vi "ble_evt_attclient_attribute_value.vi"(8 "error in (no error)":errorcluster, 11 "COM Bluegiga in":refnum<visa-resource-name>) -> (0 "error out":errorcluster, 1 "header_and_payload":u8[](array[numeric]), 2 "payload":u8[](array[numeric]), 3 "COM Bluegiga out":refnum<visa-resource-name>, 4 "attribute value":u8[](array[numeric]))   [LabVIEW 2013]
uses:
  type_def/message_class.ctl
  type_def/message_type.ctl
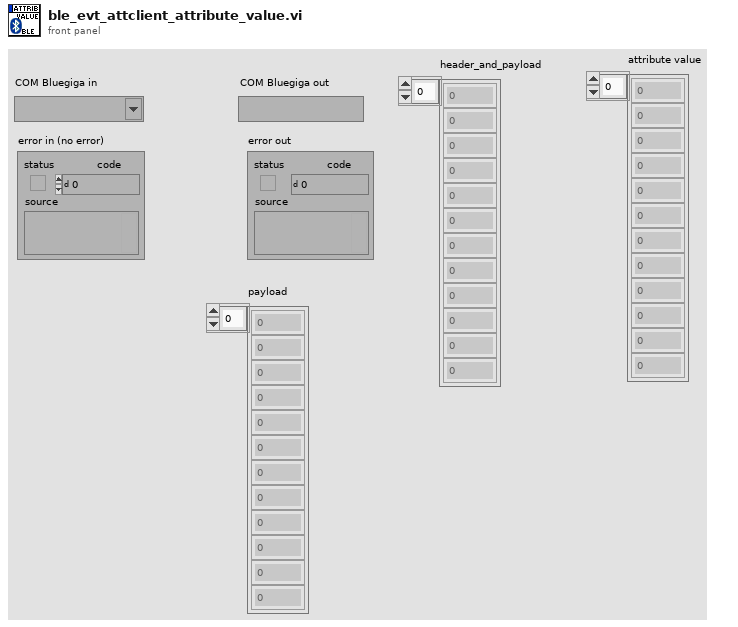
[diagram p1: front panel]
types:
  T1 = typedef "message_type.ctl" = u8
  T2 = typedef "message_class.ctl" = u8
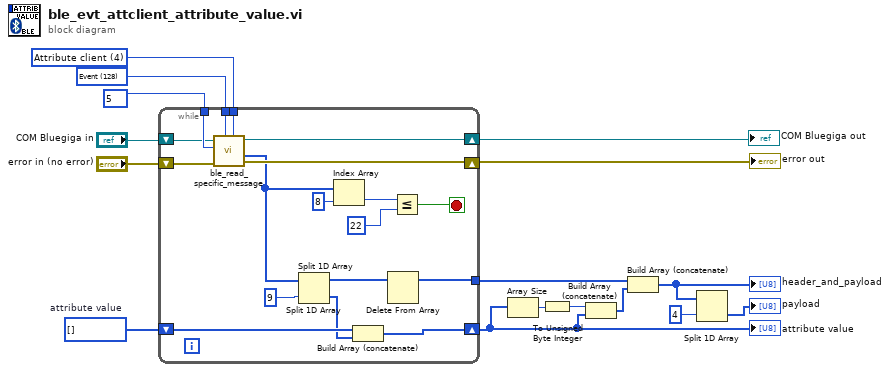
[diagram p0: block diagram]
diagram:
  w9 = u8[] []  # attribute value
  w15 = T1 128 items=["Command / Response"=0, "Event"=128] ("Message Type (Response)")
  w14 = T2 4 items=["System", "Persistent Store", "Attribute database", "Connection", "Attribute client", "Security Manager", "Generic Access Profile", "Hardware"] ("Command Class (System)")
  n1 = while {
    tunnel: u8 5 ("Message ID (0x00)") -> [w34]
    tunnel: w15 -> [w33]
    tunnel: w14 -> [w32]
    shift-right: [w23] -> w6
    shift-left: w9 -> [w24]
    shift-right: [w31] -> w13
    shift-left: "COM Bluegiga in" -> [w29]
    shift-right: [w30] -> w12
    shift-left: "error in (no error)" -> [w28]
    tunnel: [w18] -> w4
    stop <- w17 stop-if-true
    w21 = 9 ("index")
    n2 = call "ble_read_specific_message.vi"("Command Class (System)"=w32, "Message Type (Response)"=w33, "error in (no error)"=w28, "Message ID (0x00)"=w34, "COM Bluegiga in"=w29) -> ("error out"=w30:errorcluster, "full message package"=w22:u8[], "COM Bluegiga out"=w31:refnum<visa-resource-name>)  [unwired: 2 in, 2 out]
    n3 = Split 1D Array(array=w22, index=w21) -> (first subarray=w19:u8[], second subarray=w20:u8[])
    n4 = Split 1D Array(array=w22, index=w21) -> ()  [unwired: 2 out]
    n5 = Index Array(array=w22, index=8) -> (element=w26:u8)
    n6 = Build Array (concatenate)(w24, w20) -> (w23:u8[])
    n7 = Delete From Array(array=w19) -> (array with subset deleted=w18:u8[])  [unwired: 2 in, 1 out]
    n8 = Less Or Equal?(x=w26, y=u8 22) -> (x <= y?=w17:bool)
  }
  "COM Bluegiga out" <- w13
  "error out" <- w12
  "attribute value" <- w6
  n9 = Array Size(array=w6) -> (size(s)=w8:i32)
  n10 = To Unsigned Byte Integer(number=w8) -> (unsigned 8bit integer=w7:u8)
  n11 = Build Array (concatenate)(w7, w6) -> (w5:u8[])
  n12 = Build Array (concatenate)(w4, w5) -> (w3:u8[])
  "header_and_payload" <- w3
  n13 = Split 1D Array(array=w3, index=4) -> (second subarray=→"payload":u8[])  [unwired: 1 out]
